vi "3D Coordinate Conversion (Scalar).vi"(8 "conversion type":u16(ring) items=["Cartesian to Spherical", "Spherical to Cartesian", "Cartesian to Cylindrical", "Cylindrical to Cartesian", "Spherical to Cylindrical", "Cylindrical to Spherical"], 9 "axis 3":dbl, 10 "axis 2":dbl, 11 "axis 1":dbl) -> (0 "error":i32, 1 "axis 3 out":dbl, 2 "axis 2 out":dbl, 3 "axis 1 out":dbl)   [LabVIEW 2014, in "NI_AALPro.lvlib"]
doc: "Converts coordinates between the Cartesian, spherical, and cylindrical coordinate systems. Wire data to the <B>Axis 1</B> input to determine the polymorphic instance to use or manually select the instance."
uses:
  NI_AALPro.lvlib
  lvanlys.dll
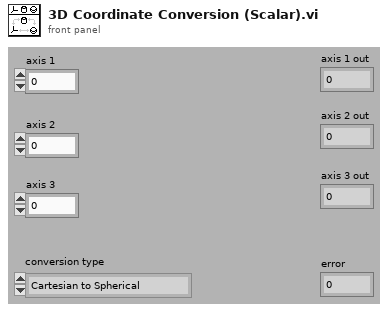
[diagram p1: front panel]
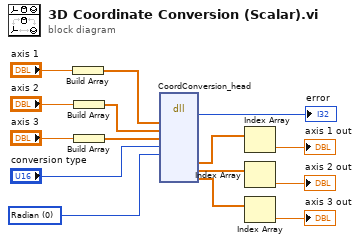
[diagram p0: block diagram]
diagram:
  w14 = u16 0 items=["Radian", "Degree"] ("unit")
  n1 = Build Array("axis 1") -> (w11:dbl[])
  n2 = Build Array("axis 2") -> (w10:dbl[])
  n3 = Build Array("axis 3") -> (w7:dbl[])
  n4 = dll-call lib="C:/Program Files (x86)/National Instruments/LabVIEW 2014/resource/lvanlys.*" fn="CoordConversion_head"("Axis1"=w11, "Axis2"=w10, "Axis3"=w7, "ConversionType"="conversion type", "unit"=w14) -> (→"error":i32, "AxisOut1"=w6:dbl[], "AxisOut2"=w4:dbl[], "AxisOut3"=w2:dbl[])  [unwired: 11 in, 2 out]
  n5 = Index Array(array=w6) -> (element=→"axis 1 out":dbl)  [unwired: 1 in]
  n6 = Index Array(array=w4) -> (element=→"axis 2 out":dbl)  [unwired: 1 in]
  n7 = Index Array(array=w2) -> (element=→"axis 3 out":dbl)  [unwired: 1 in]
